vi "Once per press.vi"(2 "In":bool) -> (0 "Out":bool)   [LabVIEW 2015]
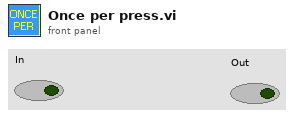
[diagram p1: front panel]
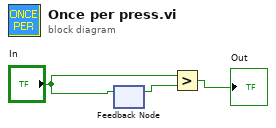
[diagram p0: block diagram]
diagram:
  n1 = feedback-in #1("In") -> ()
  n2 = feedback #1() -> (w3:bool)  [unwired: 1 in]
  n3 = Greater?(x="In", y=w3) -> (0:→"Out":bool)
